vi "State_Machine.vi"(8 "error in (no error)":errorcluster caption="entrée d'erreur (pas d'erreur)", 11 "Get_Voltage en entrée":refnum<class "Nodon_Set_Voltage_Calibration.lvclass">) -> (0 "error out":errorcluster caption="sortie d'erreur", 2 "Json_String":string, 3 "Get_Voltage en sortie":refnum<class "Nodon_Set_Voltage_Calibration.lvclass">)   [LabVIEW 2020, in "Library Test.lvlib" / "Nodon_Set_Voltage_Calibration.lvclass"]
uses:
  Nodon_Set_Voltage_Calibration.lvclass
  C:/Users/ngarcin/OneDrive - Altyor/Standard TB/Suite TB45/Class/Test/Nodon_Send_Command_UART/Nodon_Send_Command_UART.lvclass
  Commun VI/TypeDef/Variable Printable.ctl
  Nodon_Send_Command_UART.lvclass
  Commun VI/Library Commun.lvlib
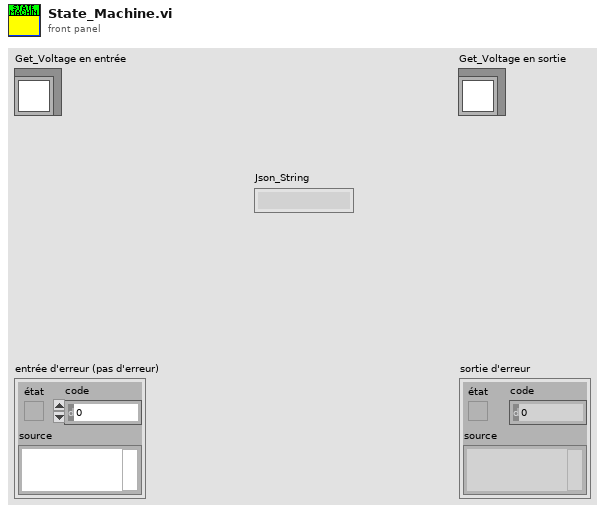
[diagram p1: front panel]
types:
  T1 = typedef "Variable Printable.ctl" = string
  T2 = enum16{"Get Variable", "Get All Variables", "Set Variable", "Delete Variable", "Delete All Variable"}
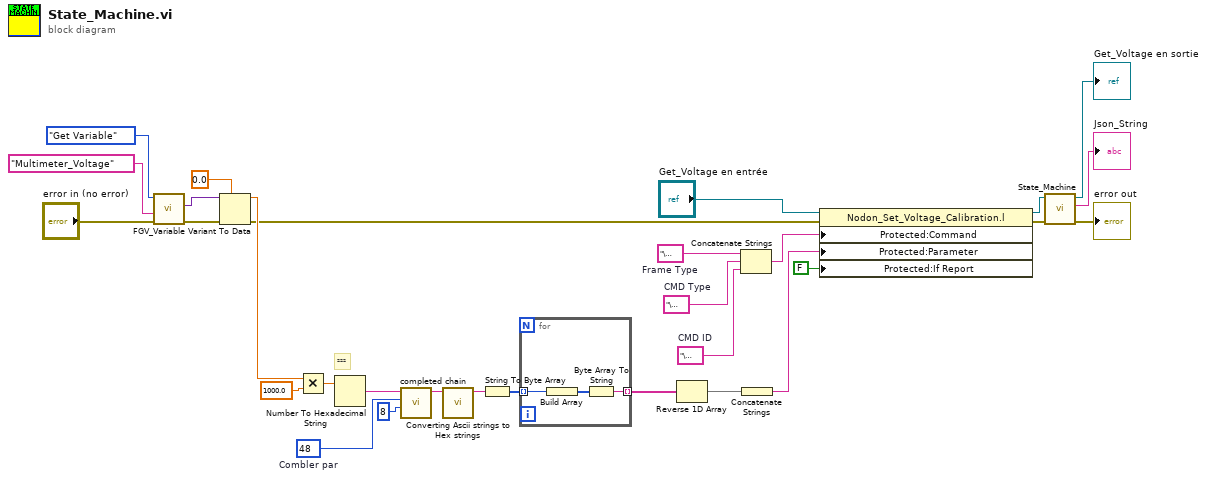
[diagram p0: block diagram]
diagram:
  w20 = u8 48  # Combler par
  w25 = "\u0000"  # Frame Type
  w24 = "\u0010"  # CMD ID
  w23 = "\u0003"  # CMD Type
  # "²²²"
  n1 = call "FGV_Variable.vi"("error in (no error)"="error in (no error)", "Variable"=T1 "Multimeter_Voltage", "Function"=T2."Get Variable") -> ("error out"=w7:errorcluster, "Data Out"=w6:variant)  [unwired: 6 in, 1 out]
  n2 = Variant To Data(error in=w7, type=0.0, Variant=w6) -> (data=w4:dbl, error out=w3:errorcluster)
  n3 = Multiply(x=w4, y=1000.0) -> (x*y=w11:dbl)
  n4 = Number To Hexadecimal String(2:w11) -> (0:w18:string)  [unwired: 1 in]
  n5 = call "completed chain.vi"("longueur"=8, "Combler par"=w20, "Chaine"=w18) -> ("chaîne"=w2:string)  [unwired: 8 in]
  n6 = call "Converting Ascii strings to Hex strings.vi"("result string"=w2) -> ("Chaîne"=w1:string)  [unwired: 10 in]
  n7 = String To Byte Array(string=w1) -> (unsigned byte array=w17:u8[])
  n8 = for {
    tunnel: [w33] -> w16 mode=indexing
    tunnel: w17 -> [w32] mode=indexing
    n9 = Build Array(w32) -> (w31:u8[])
    n10 = Byte Array To String(unsigned byte array=w31) -> (string=w33:string)
  }
  n11 = Reverse 1D Array(array=w16) -> (reversed array=w15:string[])
  n12 = Concatenate Strings(w25, w23, w24) -> (w22:string)
  n13 = Concatenate Strings(w15) -> (w14:string)
  n14 = property class="Nodon_Set_Voltage_Calibration.l"(reference="Get_Voltage en entrée", error in=w3, "Protected:Command"=w22, "Protected:Parameter"=w14, "Protected:If Report"=FALSE ("If Report")) -> (reference out=w27:refnum<class "Nodon_Set_Voltage_Calibration.lvclass">, error out=w26:errorcluster)
  n15 = call-parent "State_Machine.vi"("error in (no error)"=w26, "Send_Frame en entrée"=w27) -> ("error out"=→"error out":errorcluster, "Json_String"=→"Json_String":string, "Send_Frame en sortie"=→"Get_Voltage en sortie":refnum<class "Nodon_Set_Voltage_Calibration.lvclass">)  [unwired: 7 in]
